vi "dfd_Filter Coef to TF.vi"(8 "error out":errorcluster, 11 "filter coef":T1) -> (0 "error":errorcluster, 2 "denominator":dbl[](array[numeric]), 3 "numerator":dbl[](array[numeric]))   [LabVIEW 2017, in "NI_DigFilterLicensed.lvlib"]
uses:
  <vilib>/addons/Digital Filter Design/NI_DigFilterLicensed.lvlib
  <vilib>/addons/Digital Filter Design/_Objects.llb/DFD Filter Coef.ctl
  <vilib>/addons/Digital Filter Design/_Objects.llb/DFD Filter Structure Type Selector.ctl
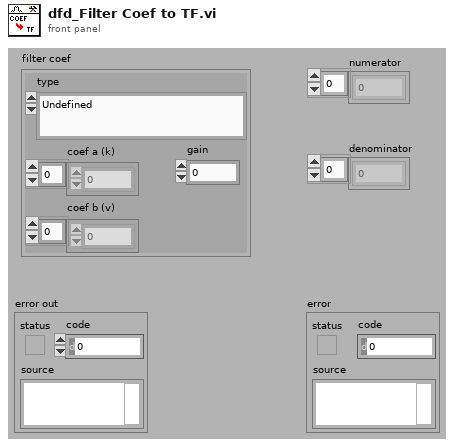
[diagram p1: front panel]
types:
  T1 = typedef "NI_DigFilterLicensed.lvlib/DFD Filter Coef.ctl" = cluster{"type":T2, "gain":dbl, "coef a (k)":dbl[], "coef b (v)":dbl[]}
  T2 = typedef "NI_DigFilterLicensed.lvlib/DFD Filter Structure Type Selector.ctl" = enum16{"Undefined", "FIR Direct Form", "FIR Direct Form Transposed", "FIR Symmetric", "FIR Antisymmetric", "IIR Direct Form I", "IIR Direct Form I Transposed", "IIR Direct Form II", "IIR Direct Form II Transposed", "IIR Cascaded Second Order Sections Form I", "IIR Cascaded Second Order Sections Form I Transposed", "IIR Cascaded Second Order Sections Form II", "IIR Cascaded Second Order Sections Form II Transposed", "Lattice Allpass (basic sections)", "Lattice Allpass (one multiplier sections)", "Lattice Allpass (normalized sections)", "Lattice AR (basic sections)", "Lattice AR (one multiplier sections)", "Lattice AR (normalized sections)", "Lattice MA (minimum phase)", "Lattice MA (maximum phase)", "Lattice ARMA (basic sections)", "Lattice ARMA (one multiplier sections)", "Lattice ARMA (normalized sections)"}
  T3 = enum16{"Basic Section", "One Multiplier Section", "Normalized Section"}
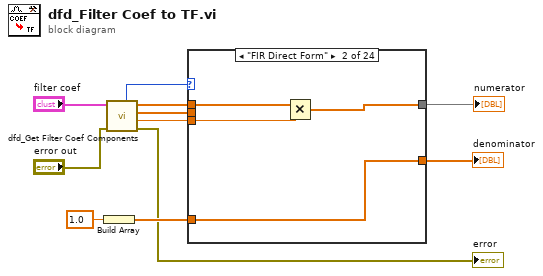
[diagram p0: block diagram]
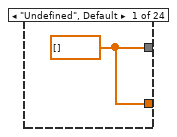
[diagram p2: hidden frame]
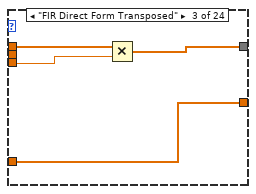
[diagram p3: hidden frame]
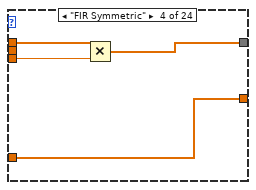
[diagram p4: hidden frame]
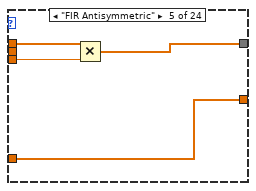
[diagram p5: hidden frame]
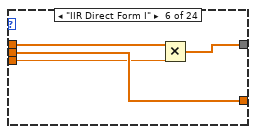
[diagram p6: hidden frame]
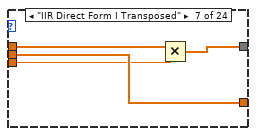
[diagram p7: hidden frame]
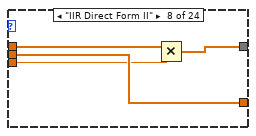
[diagram p8: hidden frame]
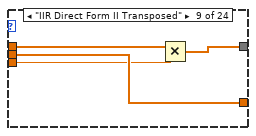
[diagram p9: hidden frame]
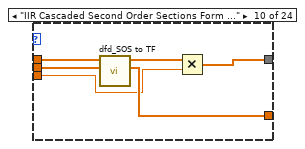
[diagram p10: hidden frame]
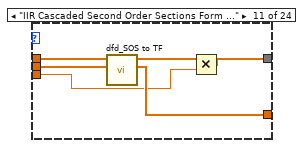
[diagram p11: hidden frame]
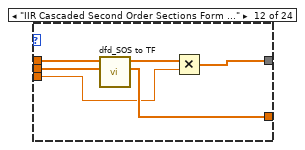
[diagram p12: hidden frame]
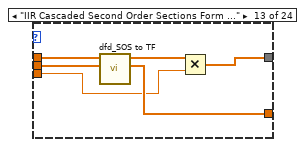
[diagram p13: hidden frame]
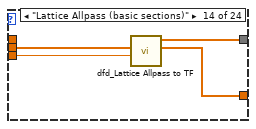
[diagram p14: hidden frame]
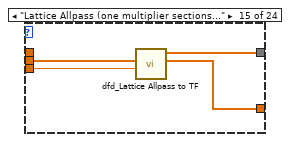
[diagram p15: hidden frame]
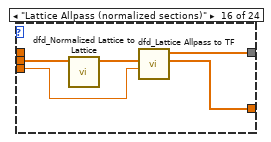
[diagram p16: hidden frame]
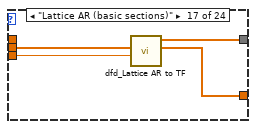
[diagram p17: hidden frame]
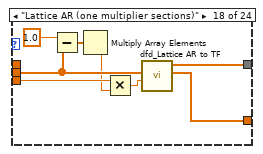
[diagram p18: hidden frame]
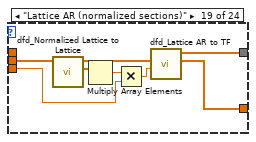
[diagram p19: hidden frame]
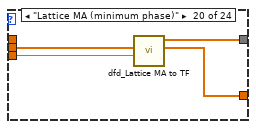
[diagram p20: hidden frame]
diagram:
  n1 = Build Array(1.0 ("element")) -> (w8:dbl[])
  n2 = call <vilib>:"dfd_Get Filter Coef Components.vi"("error in (no error)"="error out", "filter coef"="filter coef") -> ("error out"=→"error":errorcluster, "gain"=w2:dbl, "coef a (k)"=w6:dbl[], "coef b (v)"=w7:dbl[], "type"=w5:T2)  [unwired: 5 out]
  n3 = case shown="\"FIR Direct Form\"" w5 {
    tunnel: w7 -> [_ w15 w19 w22 w26 w30 w36 w40 w44 w50 w56 w62 w68 _ _ _ _ _ _ _ _ w114 w122 w128]
    tunnel: w6 -> [_ _ _ _ _ w32 w35 w39 w43 w49 w55 w61 w67 w70 w74 w79 w84 w91 w100 w102 w106 w113 w123 w127]
    tunnel: [w12 w14 w18 w23 w27 w31 w34 w38 w42 w46 w53 w59 w65 w72 w76 w81 w83 w89 w97 w105 w107 w112 w120 w126] -> w1
    tunnel: [w12 w16 w20 w24 w28 w32 w35 w39 w43 w47 w54 w60 w66 w71 w75 w80 w85 w93 w101 w104 w109 w116 w124 w130] -> w4
    tunnel: w8 -> [_ w16 w20 w24 w28 _ _ _ _ _ _ _ _ _ _ _ _ _ _ _ _ _ _ _]
    tunnel: w2 -> [_ w13 w17 w21 w25 w29 w33 w37 w41 w45 w51 w57 w63 w69 w73 w77 w82 w87 w95 w103 w108 w111 w118 w125]
    frame "Undefined", Default {
      w12 = dbl[] [] ("numerator")
    }
    frame "FIR Direct Form" {
      n4 = Multiply(x=w15, y=w13) -> (x*y=w14:dbl[])
    }
    frame "FIR Direct Form Transposed" {
      n5 = Multiply(x=w19, y=w17) -> (x*y=w18:dbl[])
    }
    frame "FIR Symmetric" {
      n6 = Multiply(x=w22, y=w21) -> (x*y=w23:dbl[])
    }
    frame "FIR Antisymmetric" {
      n7 = Multiply(x=w26, y=w25) -> (x*y=w27:dbl[])
    }
    frame "IIR Direct Form I" {
      n8 = Multiply(x=w30, y=w29) -> (x*y=w31:dbl[])
    }
    frame "IIR Direct Form I Transposed" {
      n9 = Multiply(x=w36, y=w33) -> (x*y=w34:dbl[])
    }
    frame "IIR Direct Form II" {
      n10 = Multiply(x=w40, y=w37) -> (x*y=w38:dbl[])
    }
    frame "IIR Direct Form II Transposed" {
      n11 = Multiply(x=w44, y=w41) -> (x*y=w42:dbl[])
    }
    frame "IIR Cascaded Second Order Sections Form I" {
      n12 = call <vilib>:"dfd_SOS to TF.vi"("SOS reverse coefficients"=w49, "SOS forward coefficients"=w50) -> ("denominator"=w47:dbl[], "numerator"=w48:dbl[])  [unwired: 8 out]
      n13 = Multiply(x=w48, y=w45) -> (x*y=w46:dbl[])
    }
    frame "IIR Cascaded Second Order Sections Form I Transposed" {
      n14 = call <vilib>:"dfd_SOS to TF.vi"("SOS reverse coefficients"=w55, "SOS forward coefficients"=w56) -> ("denominator"=w54:dbl[], "numerator"=w52:dbl[])  [unwired: 8 out]
      n15 = Multiply(x=w52, y=w51) -> (x*y=w53:dbl[])
    }
    frame "IIR Cascaded Second Order Sections Form II" {
      n16 = call <vilib>:"dfd_SOS to TF.vi"("SOS reverse coefficients"=w61, "SOS forward coefficients"=w62) -> ("denominator"=w60:dbl[], "numerator"=w58:dbl[])  [unwired: 8 out]
      n17 = Multiply(x=w58, y=w57) -> (x*y=w59:dbl[])
    }
    frame "IIR Cascaded Second Order Sections Form II Transposed" {
      n18 = call <vilib>:"dfd_SOS to TF.vi"("SOS reverse coefficients"=w67, "SOS forward coefficients"=w68) -> ("denominator"=w66:dbl[], "numerator"=w64:dbl[])  [unwired: 8 out]
      n19 = Multiply(x=w64, y=w63) -> (x*y=w65:dbl[])
    }
    frame "Lattice Allpass (basic sections)" {
      n20 = call <vilib>:"dfd_Lattice Allpass to TF.vi"("gain"=w69, "k [1~M]"=w70) -> ("denominator"=w71:dbl[], "numerator"=w72:dbl[])  [unwired: 1 in, 7 out]
    }
    frame "Lattice Allpass (one multiplier sections)" {
      n21 = call <vilib>:"dfd_Lattice Allpass to TF.vi"("gain"=w73, "k [1~M]"=w74) -> ("denominator"=w75:dbl[], "numerator"=w76:dbl[])  [unwired: 1 in, 7 out]
    }
    frame "Lattice Allpass (normalized sections)" {
      n22 = call <vilib>:"dfd_Normalized Lattice to Lattice.vi"("k & ^k"=w79) -> ("k [M~1]"=w78:dbl[])  [unwired: 10 out]
      n23 = call <vilib>:"dfd_Lattice Allpass to TF.vi"("gain"=w77, "k [1~M]"=w78) -> ("denominator"=w80:dbl[], "numerator"=w81:dbl[])  [unwired: 1 in, 7 out]
    }
    frame "Lattice AR (basic sections)" {
      n24 = call <vilib>:"dfd_Lattice AR to TF.vi"("gain"=w82, "k [1~M]"=w84) -> ("denominator"=w85:dbl[], "numerator"=w83:dbl[])  [unwired: 1 in, 7 out]
    }
    frame "Lattice AR (one multiplier sections)" {
      n25 = Subtract(x=1.0, y=w91) -> (x-y=w90:dbl[])
      n26 = Multiply Array Elements(1:w90) -> (0:w86:dbl)
      n27 = Multiply(x=w87, y=w86) -> (x*y=w88:dbl)
      n28 = call <vilib>:"dfd_Lattice AR to TF.vi"("gain"=w88, "k [1~M]"=w91) -> ("denominator"=w93:dbl[], "numerator"=w89:dbl[])  [unwired: 1 in, 7 out]
    }
    frame "Lattice AR (normalized sections)" {
      n29 = call <vilib>:"dfd_Normalized Lattice to Lattice.vi"("k & ^k"=w100) -> ("^k [M~1]"=w98:dbl[], "k [M~1]"=w99:dbl[])  [unwired: 9 out]
      n30 = Multiply Array Elements(1:w98) -> (0:w96:dbl)
      n31 = Multiply(x=w96, y=w95) -> (x*y=w94:dbl)
      n32 = call <vilib>:"dfd_Lattice AR to TF.vi"("gain"=w94, "k [1~M]"=w99) -> ("denominator"=w101:dbl[], "numerator"=w97:dbl[])  [unwired: 1 in, 7 out]
    }
    frame "Lattice MA (minimum phase)" {
      n33 = call <vilib>:"dfd_Lattice MA to TF.vi"("gain"=w103, "k [1~M]"=w102) -> ("denominator"=w104:dbl[], "numerator"=w105:dbl[])  [unwired: 1 in, 7 out]
    }
    frame "Lattice MA (maximum phase)" {
      n34 = call <vilib>:"dfd_Lattice MA to TF.vi"("gain"=w108, "k [1~M]"=w106) -> ("denominator"=w109:dbl[], "numerator"=w110:dbl[])  [unwired: 1 in, 7 out]
      n35 = Reverse 1D Array(array=w110) -> (reversed array=w107:dbl[])
    }
    frame "Lattice ARMA (basic sections)" {
      n36 = call <vilib>:"dfd_Lattice ARMA to TF.vi"("section type"=T3."Basic Section", "k"=w113, "v"=w114) -> ("denominator"=w116:dbl[], "numerator"=w117:dbl[])  [unwired: 7 out]
      n37 = Multiply(x=w117, y=w111) -> (x*y=w112:dbl[])
    }
    frame "Lattice ARMA (one multiplier sections)" {
      n38 = call <vilib>:"dfd_Lattice ARMA to TF.vi"("section type"=T3."One Multiplier Section", "k"=w123, "v"=w122) -> ("denominator"=w124:dbl[], "numerator"=w119:dbl[])  [unwired: 7 out]
      n39 = Multiply(x=w119, y=w118) -> (x*y=w120:dbl[])
    }
    frame "Lattice ARMA (normalized sections)" {
      n40 = call <vilib>:"dfd_Lattice ARMA to TF.vi"("section type"=T3."Normalized Section", "k"=w127, "v"=w128) -> ("denominator"=w130:dbl[], "numerator"=w131:dbl[])  [unwired: 7 out]
      n41 = Multiply(x=w131, y=w125) -> (x*y=w126:dbl[])
    }
  }
  "denominator" <- w4
  "numerator" <- w1
